vi "Publish UI Closed.vi"(8 "error in":errorcluster, 10 "Closed":bool, 11 "Flex  Dialog (Actor) in":refnum<class "Flex Dialog (Actor).lvclass">) -> (0 "error out":errorcluster, 3 "Flex  Dialog (Actor) out":refnum<class "Flex Dialog (Actor).lvclass">)   [LabVIEW 2014, in "Flex UI Dialog (Actor).lvlib" / "Flex Dialog (Actor).lvclass"]
uses:
  Flex Dialog (Actor).lvclass
  Flex Dialog (Actor).lvclass/Flex Dialog (Actor).ctl
  <vilib>/East West Architects/MVC Subscription/Subscription/MVC Subscription.lvclass
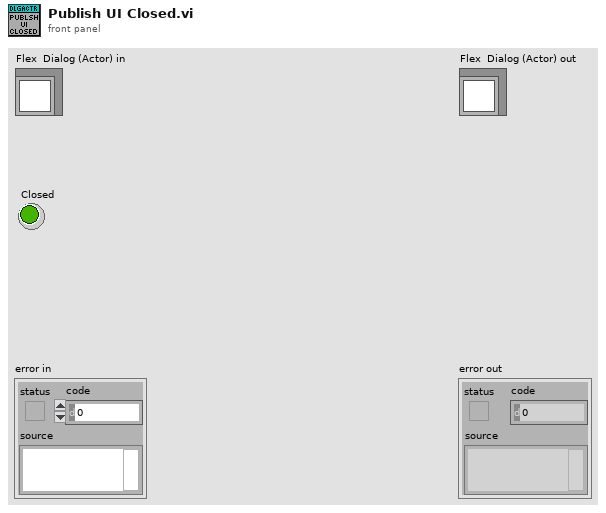
[diagram p1: front panel]
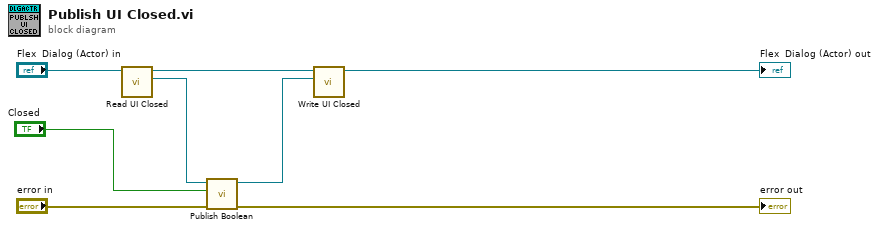
[diagram p0: block diagram]
diagram:
  n1 = call "Read UI Closed.vi"("Flex  Dialog (Actor) in"="Flex  Dialog (Actor) in") -> ("Subscriptions.UI Closed"=w1:refnum<class "MVC Subscription.lvclass">, "Flex  Dialog (Actor) out"=w6:refnum<class "Flex Dialog (Actor).lvclass">)  [unwired: 9 in]
  n2 = call <vilib>:"Publish Boolean.vi"("error in (no error)"="error in", "Boolean"="Closed", "MVC Subscription in"=w1) -> ("error out"=→"error out":errorcluster, "MVC Subscription out"=w3:refnum<class "MVC Subscription.lvclass">)  [unwired: 7 in]
  n3 = call "Write UI Closed.vi"("Subscriptions.UI Closed"=w3, "Flex  Dialog (Actor) in"=w6) -> ("Flex  Dialog (Actor) out"=→"Flex  Dialog (Actor) out":refnum<class "Flex Dialog (Actor).lvclass">)  [unwired: 9 in]
